vi "main_magneto_ard.vi"() -> ()   [LabVIEW 2012]
uses:
  <vilib>/LabVIEW Interface for Arduino/LabVIEW Interface for Arduino.lvlib
  HMC5883L.lvclass
panel:
  in  "stop":bool
  out "Raw.ZAxis":i16
  out "Raw.YAxis":i16
  out "Raw.XAxis":i16
  out "Scaled.ZAxis":sgl
  out "Scaled.YAxis":sgl
  out "Scaled.XAxis":sgl
  out "heading":dbl
  out "headingDegrees":dbl
  out "HMC5883L out":refnum<class "HMC5883L.lvclass">
  in  "mode":T1(ring)
  in  "Gauss":T2(ring)
  in  "HMC5883L":refnum<class "HMC5883L.lvclass">
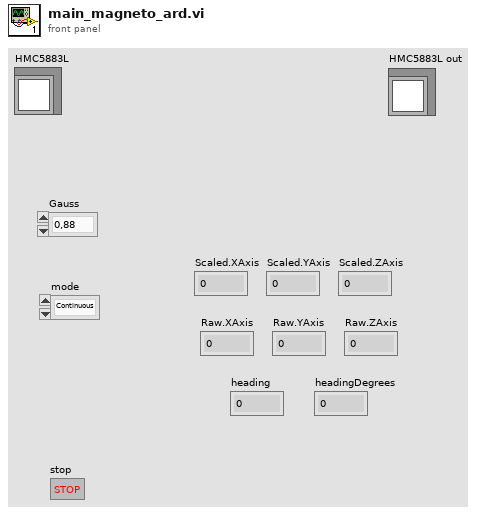
[diagram p1: front panel]
types:
  T1 = enum16{"Continuous", "SingleShot", "NoDefined", "Idle"}
  T2 = enum8{"0,88", "1,30", "1,90", "2,50", "4,00", "4,70", "5,60", "8,10"}
  T3 = typedef "LabVIEW Interface for Arduino.lvlib/Arduino Resource.ctl" = cluster{"VISA resource":refnum<visa-resource-name>, "Board Type":T4, "Connection Type":enum8{"USB / Serial"}, "Bytes Per Packet (15)":u8}
  T4 = typedef "LabVIEW Interface for Arduino.lvlib/Board Type.ctl" = enum16{"Uno", "Dimuelanove w/Atmega 328", "Mega 2560"}
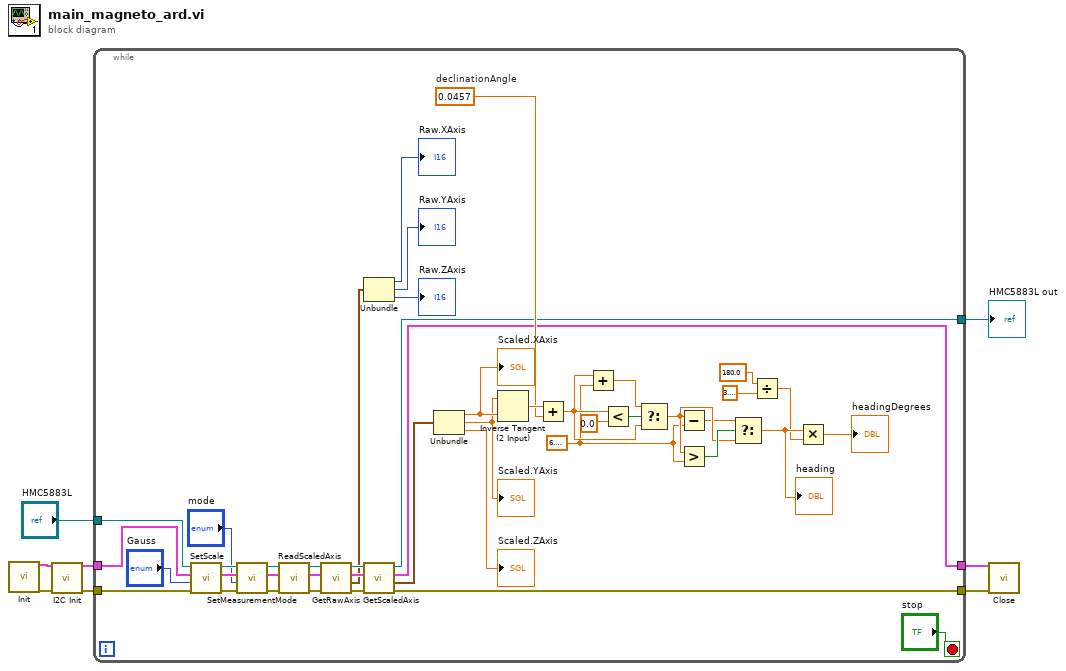
[diagram p0: block diagram]
diagram:
  n1 = call <vilib>:"Init.vi"() -> ("Arduino Resource"=w8:T3, "error out"=w7:errorcluster)  [unwired: 18 in]
  n2 = call <vilib>:"I2C Init.vi"("Arduino Resource"=w8, "error in"=w7) -> ("Arduino Resource"=w5:T3, "error out"=w4:errorcluster)  [unwired: 12 in]
  n3 = while {
    tunnel: "HMC5883L" -> [w52]
    tunnel: w5 -> [w51]
    tunnel: w4 -> [w50]
    tunnel: [w28] -> w3
    tunnel: [w27] -> w2
    tunnel: [w26] -> w1
    stop <- "stop" stop-if-true
    w37 = 0.0457  # declinationAngle
    w30 = 6.283185307179586
    n4 = call-dynamic "SetScale.vi"("error in (no error)"=w50, "Gauss"="Gauss", "Arduino Resource In"=w51, "HMC5883L in"=w52) -> ("error out"=w46:errorcluster, "Arduino Resource Out"=w47:T3, "HMC5883L out"=w48:refnum<class "HMC5883L.lvclass">)  [unwired: 5 in]
    n5 = call-dynamic "SetMeasurementMode.vi"("error in (no error)"=w46, "mode"="mode", "Arduino Resource In"=w47, "HMC5883L in"=w48) -> ("error out"=w39:errorcluster, "Arduino Resource Out"=w40:T3, "HMC5883L out"=w41:refnum<class "HMC5883L.lvclass">)  [unwired: 5 in]
    n6 = call-dynamic "ReadScaledAxis.vi"("error in (no error)"=w39, "Arduino Resource In"=w40, "HMC5883L in"=w41) -> ("error out"=w16:errorcluster, "Arduino Resource out"=w18:T3, "HMC5883L out"=w20:refnum<class "HMC5883L.lvclass">)  [unwired: 6 in]
    n7 = call-dynamic "GetRawAxis.vi"("error in (no error)"=w16, "Arduino Resource In"=w18, "HMC5883L in"=w20) -> ("error out"=w15:errorcluster, "MagnetometerRaw"=w14:cluster{"XAxis":i16, "YAxis":i16, "ZAxis":i16}, "Arduino Resource out"=w17:T3, "HMC5883L out"=w19:refnum<class "HMC5883L.lvclass">)  [unwired: 5 in]
    n8 = Unbundle(w14) -> ("XAxis"=→"Raw.XAxis":i16, "YAxis"=→"Raw.YAxis":i16, "ZAxis"=→"Raw.ZAxis":i16)
    n9 = call-dynamic "GetScaledAxis.vi"("error in (no error)"=w15, "Arduino Resource In"=w17, "HMC5883L in"=w19) -> ("error out"=w28:errorcluster, "MagnetometerScaled"=w44:cluster{"XAxis":sgl, "YAxis":sgl, "ZAxis":sgl}, "Arduino Resource out"=w27:T3, "HMC5883L out"=w26:refnum<class "HMC5883L.lvclass">)  [unwired: 5 in]
    n10 = Unbundle(w44) -> ("XAxis"=w43:sgl, "YAxis"=w42:sgl, "ZAxis"=→"Scaled.ZAxis":sgl)
    "Scaled.XAxis" <- w43
    "Scaled.YAxis" <- w42
    n11 = Inverse Tangent (2 Input)(1:w43, 2:w42) -> (0:w38:sgl)
    n12 = Add(x=w38, y=w37) -> (x+y=w33:dbl)
    n13 = Add(x=w33, y=w30) -> (x+y=w34:dbl)
    n14 = Less?(x=w33, y=0.0) -> (x < y?=w36:bool)
    n15 = Select(t=w34, s=w36, f=w33) -> (s? t:f=w31:dbl)
    n16 = Subtract(x=w31, y=w30) -> (x-y=w29:dbl)
    n17 = Greater?(x=w31, y=w30) -> (0:w32:bool)
    n18 = Select(t=w29, s=w32, f=w31) -> (s? t:f=w23:dbl)
    "heading" <- w23
    n19 = Divide(x=180.0, y=3.141592653589793) -> (x/y=w22:dbl)
    n20 = Multiply(x=w23, y=w22) -> (x*y=→"headingDegrees":dbl)
  }
  "HMC5883L out" <- w1
  n21 = call <vilib>:"Close.vi"("Arduino Resource"=w2, "error in"=w3) -> ()  [unwired: 13 in, 1 out]
